vi "Deselect All groups.vi"(11 "Deselect all groups":bool=TRUE) -> (0 "error out":errorcluster)   [LabVIEW 2020]
uses:
  Global variables/gl_Functional Imaging-Global variables.vi
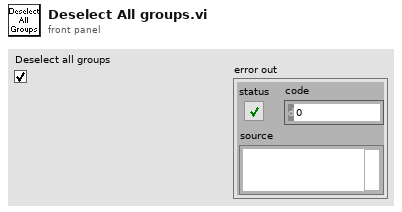
[diagram p1: front panel]
types:
  T1 = typedef "Functional Imging UI Refs.ctl" = cluster{"Menu ref":refnum<k9>, "Image control":refnum<vi>, "VI ref":refnum<vi>, "XGrapher":refnum<vi>, "Smoothing":refnum<vi>, "POI Averaging":refnum<vi>, "Normalize":refnum<vi>, "POI data points in each trial":refnum<vi>, "Channel":refnum<vi>, "Experiment data folder path":refnum<vi>, "[ROI vis]":refnum<vi>, "[Groups] visbl":T2, "Group Name":refnum<vi>, "POI index":refnum<vi>, "Trial No.":refnum<vi>, "Intensity Zoom":refnum<vi>, "Trial Cursor Enabled":refnum<vi>, "Number of Trials (ind 1)":refnum<vi>, "Number of Trials (ind 2)":refnum<vi>, "MiniScans Available":refnum<vi>, "POI Available":refnum<vi>, "Defer graph updates":refnum<vi>, "Waveform selector":refnum<vi>, "#of selected POI":refnum<vi>, "#of selected MiniScans":refnum<vi>, "#of selected groups":refnum<vi>, "Max Z-Projection":refnum<vi>, "Z-Plane Selector":refnum<vi>, "Index of miniscan point to visualise":refnum<vi>, "ROI vis. mode":refnum<vi>, "Total # of points":refnum<vi>, "Index of group clicked on":refnum<vi>, "Pane 1":refnum<vi>, "Pane 2":refnum<vi>, "Pane 3":refnum<vi>, "Pane 4":refnum<vi>, "Pane 5":refnum<vi>, "Pane 6":refnum<vi>, "Deselect all ROI":refnum<vi>, "Deselect all groups":refnum<vi>}
  T2 = typedef "Groups array referecne.ctl" = refnum<vi>
  T3 = typedef "Group sel cluster.ctl" = cluster{"Group number":string, "Group Name":string, "Visibility":bool, "Highlight":bool}
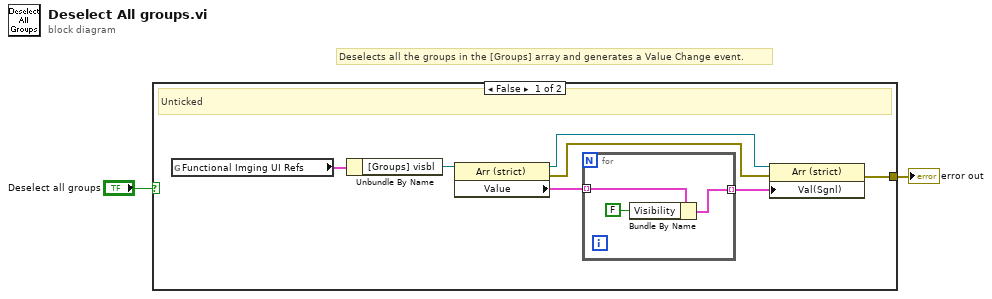
[diagram p0: block diagram]
diagram:
  # "Deselects all the groups in the [Groups] array and generates a Value Change event."
  n1 = case shown="False" "Deselect all groups" {
    tunnel: [w3 _] -> w2
    frame False {
      # "Unticked"
      n2 = global read "gl_Functional Imaging-Global variables.vi" "Functional Imging UI Refs"() -> (w4:T1)
      n3 = Unbundle By Name(w4) -> ("[Groups] visbl"=w5:T2)
      n4 = property class="Arr (strict)"(reference=w5) -> (reference out=w7:T2, error out=w9:errorcluster, "Value"=w6:T3[])  [unwired: 1 in]
      n5 = for {
        tunnel: w6 -> [w12] mode=indexing
        tunnel: [w10] -> w8 mode=indexing
        n6 = Bundle By Name(cluster=w12, "Visibility"=FALSE) -> (w10:T3)
      }
      n7 = property class="Arr (strict)"(reference=w7, error in=w9, "Val(Sgnl)"=w8) -> (error out=w3:errorcluster)  [unwired: 1 out]
    }
    frame True {
    }
  }
  "error out" <- w2
